vi "RX.vi"() -> ()   [LabVIEW 2013]
uses:
  <instrlib>/niUSRP/niUSRP Fetch Rx Data (CDB WDT).vi
  <vilib>/express/express analysis/Spectral/Block/exnSpectralBlock spectral measurements RMS poly.vi
  <vilib>/express/express analysis/Spectral/Block/exnSpectralBlock spectral measurements RMS WFM.vi
  <vilib>/express/express analysis/Spectral/XNode/ExpressSpectralMeasurementsBlockNode.xnode
panel:
  in  "number of samples":i64=100000
  out "Spectrum":cluster{"f0":dbl, "df":dbl, "magnitude":dbl[]}(graph)={"f0"=0.0, "df"=2.0, "magnitude"=array[50000 elements]}
  out "Waveform":waveform(dbl)[](graph)
  in  "active antenna":string
  out "coerced gain":dbl format="%#_6f"
  out "coerced carrier frequency":dbl=100000.0 format="%#_6p"
  out "coerced IQ rate":dbl=100000.0 format="%#_6p"
  in  "gain":dbl format="%#_6f"
  in  "carrier frequency":dbl=100000.0 format="%#_6p"
  in  "IQ rate":dbl=100000.0 format="%#_6p"
  in  "device names":refnum<k15>="192.168.10.3"
  out "error out":errorcluster
  in  "stop":bool
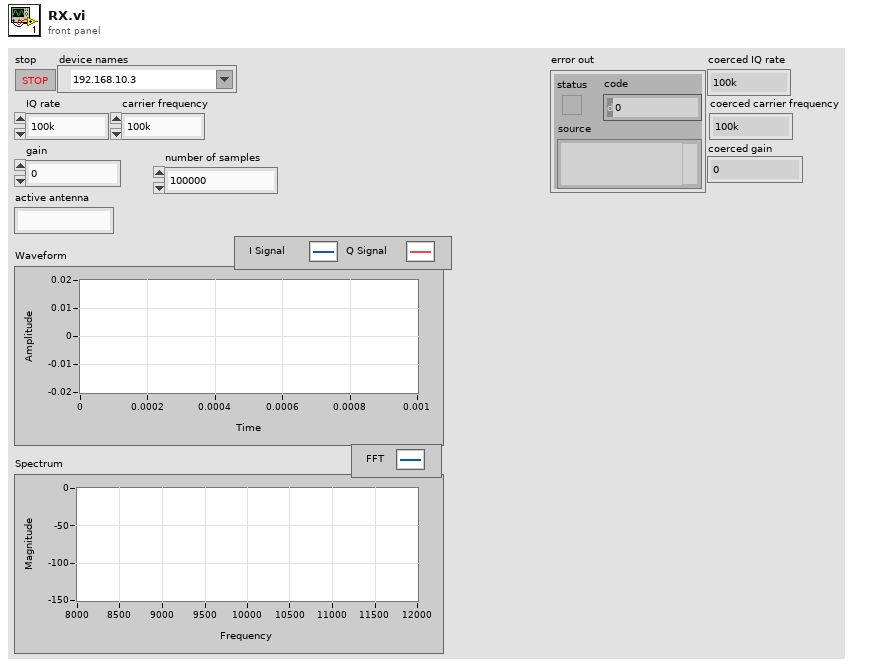
[diagram p1: front panel]
types:
  T1 = cluster{"averaging mode":u16, "weighting mode":u16, "number of averages":u32}
  T2 = cluster{"dB On (F)":bool, "unwrap phase (F)":bool, "convert to degree (F)":bool}
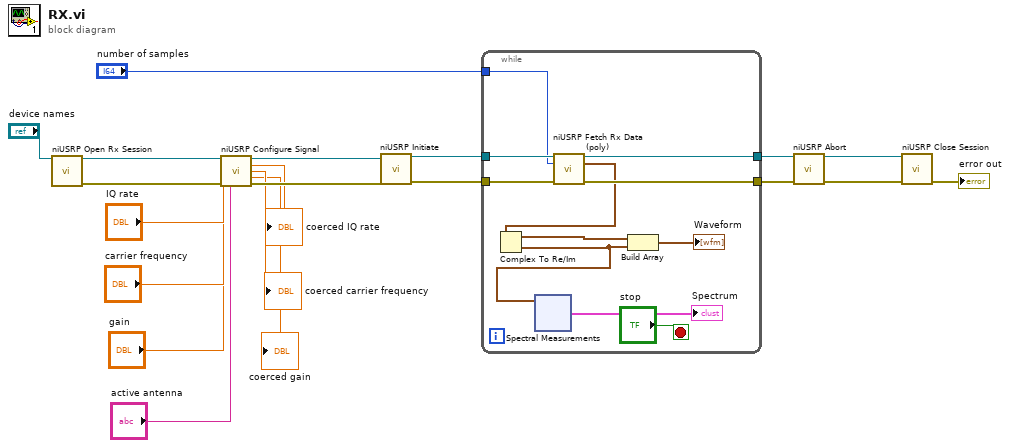
[diagram p0: block diagram]
diagram:
  n1 = call <instrlib>:"niUSRP Open Rx Session.vi"("device names"="device names") -> ("session handle out"=w20:refnum<k15>, "error out"=w15:errorcluster)  [unwired: 13 in]
  n2 = call <instrlib>:"niUSRP Configure Signal.vi"("session handle"=w20, "IQ rate"="IQ rate", "carrier frequency"="carrier frequency", "gain"="gain", "error in (no error)"=w15, "active antenna"="active antenna") -> ("session handle out"=w19:refnum<k15>, "coerced IQ rate"=→"coerced IQ rate":dbl, "coerced carrier frequency"=→"coerced carrier frequency":dbl, "coerced gain"=→"coerced gain":dbl, "error out"=w14:errorcluster)  [unwired: 5 in]
  n3 = call <instrlib>:"niUSRP Initiate.vi"("session handle"=w19, "error in (no error)"=w14) -> ("session handle out"=w18:refnum<k15>, "error out"=w13:errorcluster)  [unwired: 12 in]
  n4 = while {
    tunnel: w18 -> [w30]
    tunnel: [w29] -> w17
    tunnel: w13 -> [w28]
    tunnel: [w27] -> w12
    tunnel: "number of samples" -> [w21]
    stop <- "stop" stop-if-true
    n5 = call-poly <instrlib>:"niUSRP Fetch Rx Data (poly).vi"("session handle"=w30, "number of samples"=w21, "error in (no error)"=w28) -> ("session handle out"=w29:refnum<k15>, "data"=w22:waveform(cdb), "error out"=w27:errorcluster)  [unwired: 9 in, 1 out]
    n6 = Complex To Re/Im(x + iy=w22) -> (x=w26:waveform(dbl), y=w24:waveform(dbl))
    n7 = xnode "Spectral Measurements"("Signals"=w24) -> ("FFT - (RMS)"=→"Spectrum":cluster{"f0":dbl, "df":dbl, "magnitude":dbl[]})  [unwired: 1 in, 2 out]
    n8 = Build Array(w26, w24) -> (→"Waveform":waveform(dbl)[])
  }
  n9 = call <instrlib>:"niUSRP Abort.vi"("session handle"=w17, "error in (no error)"=w12) -> ("session handle out"=w16:refnum<k15>, "error out"=w11:errorcluster)  [unwired: 12 in]
  n10 = call <instrlib>:"niUSRP Close Session.vi"("session handle"=w16, "error in (no error)"=w11) -> ("error out"=→"error out":errorcluster)  [unwired: 13 in]
